vi "(A) Test (SubVI).vi"(0 "References IN":T1, 11 "Initialize":bool, 13 "Strain OK?":bool=TRUE) -> (8 "STOP-PROGRAM":bool, 15 "Step Number":i32)   [LabVIEW 2010]
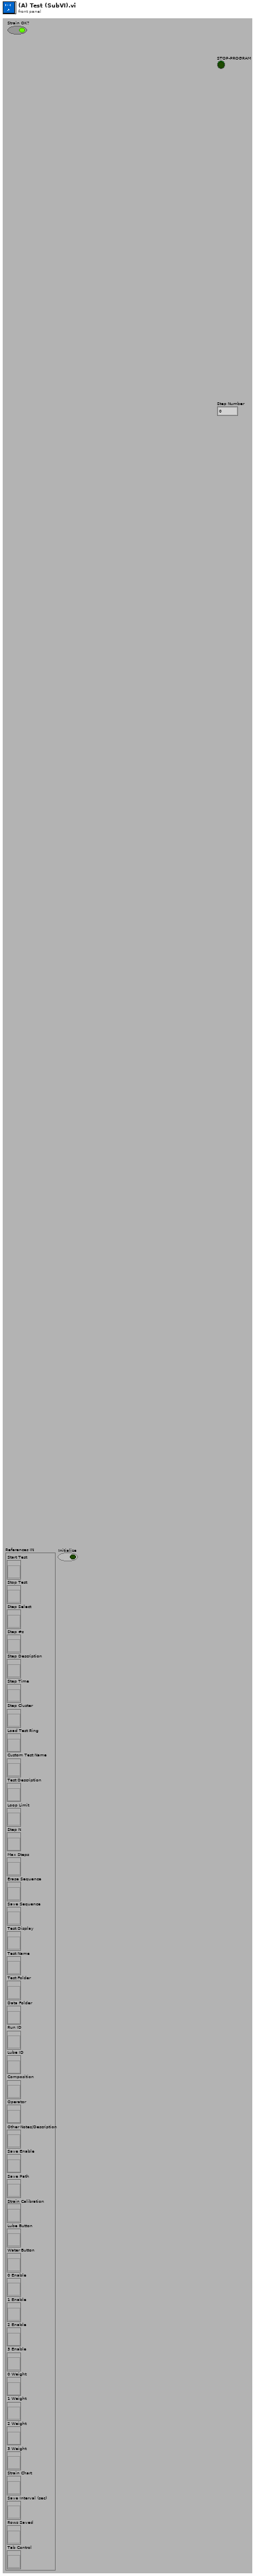
[diagram p1: front panel]
types:
  T1 = cluster{"Start Test":refnum<vi>, "Stop Test":refnum<vi>, "Step Select":refnum<vi>, "Step #s":refnum<vi>, "Step Description":refnum<vi>, "Step Time":refnum<vi>, "Step Cluster":refnum<vi>, "Load Test Ring":refnum<vi>, "Custom Test Name":refnum<vi>, "Test Description":refnum<vi>, "Loop Limit":refnum<vi>, "Step N":refnum<vi>, "Max Steps":refnum<vi>, "Erase Sequence":refnum<vi>, "Save Sequence":refnum<vi>, "Test Display":refnum<vi>, "Test Name":refnum<vi>, "Test Folder":refnum<vi>, "Data Folder":refnum<vi>, "Run ID":refnum<vi>, "Lube ID":refnum<vi>, "Composition":refnum<vi>, "Operator":refnum<vi>, "Other Notes/Description":refnum<vi>, "Save Enable":refnum<vi>, "Save Path":refnum<vi>, "Strain Calibration":refnum<vi>, "Lube Button":refnum<vi>, "Water Button":refnum<vi>, "0 Enable":refnum<vi>, "1 Enable":refnum<vi>, "2 Enable":refnum<vi>, "3 Enable":refnum<vi>, "0 Weight":refnum<vi>, "1 Weight":refnum<vi>, "2 Weight":refnum<vi>, "3 Weight":refnum<vi>, "Strain Chart":refnum<vi>, "Save Interval (sec)":refnum<vi>, "Rows Saved":refnum<vi>, "Tab Control":refnum<vi>}
  T2 = cluster{"Step Time Unit":u16, "Step End Action":u16, "Relay1":bool, "Relay2":bool}[]
  T3 = cluster{"Step Description":string, "Step Time Target":dbl, "Step Time Unit":u16, "Step End Action":u16}
  T4 = cluster{"Step Time Unit":u16, "Step End Action":u16, "Relay1":bool, "Relay2":bool}
  T5 = enum8{"Enabled", "Disabled", "Disabled and Grayed Out"}
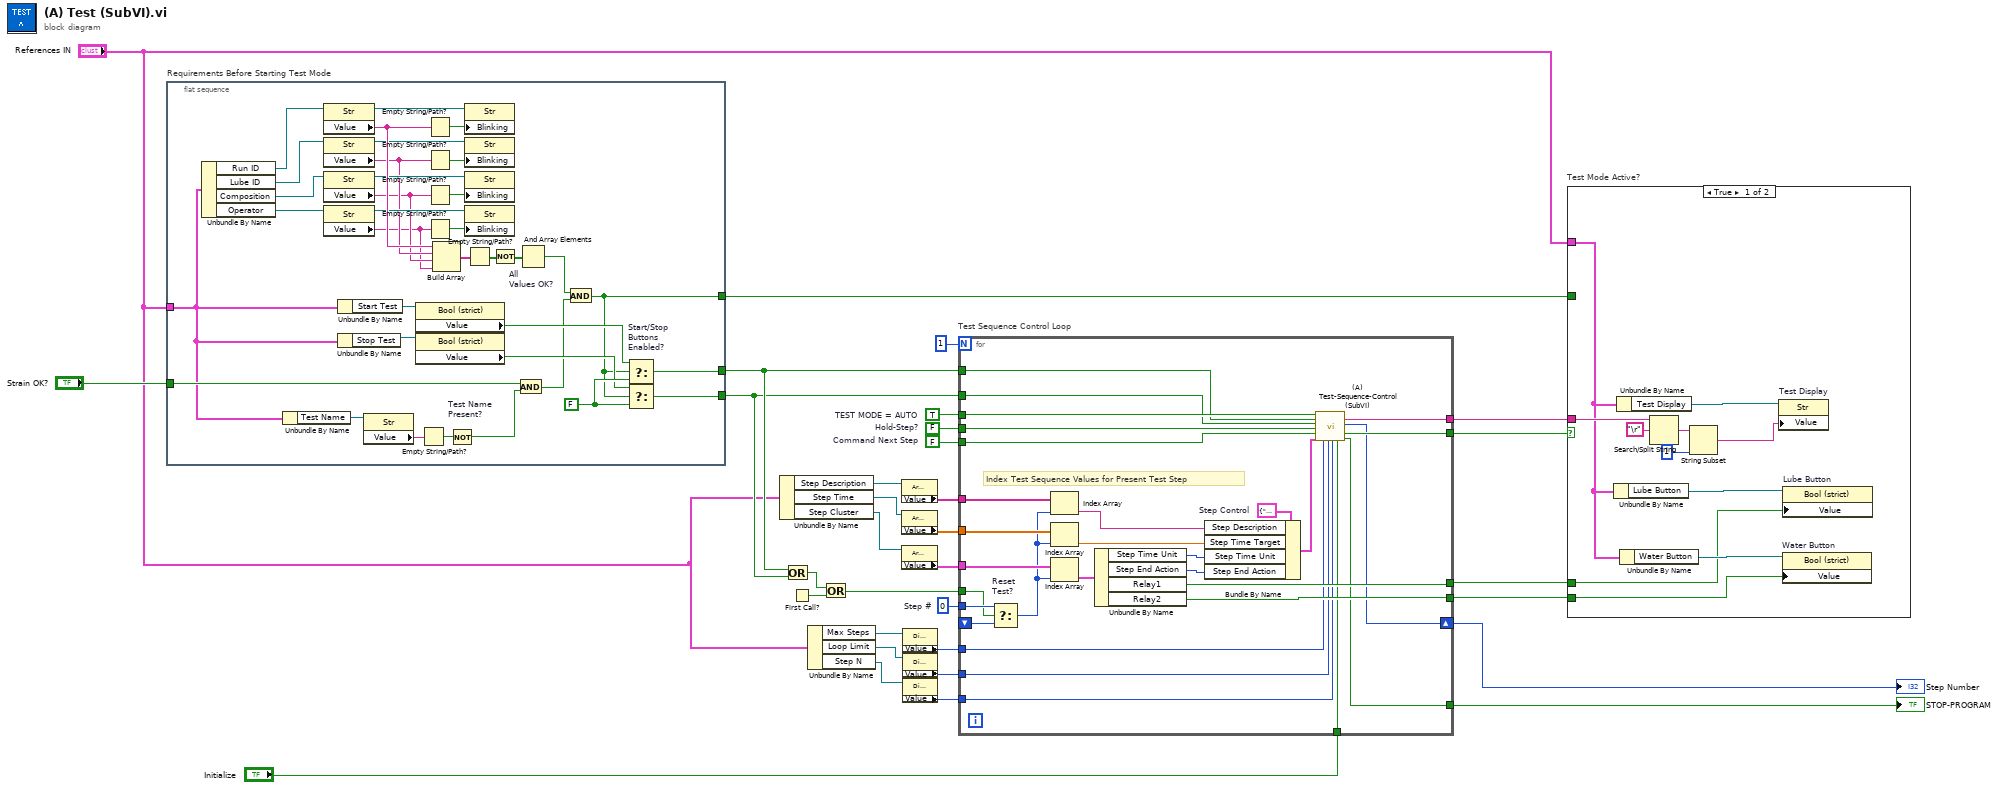
[diagram p0: block diagram]
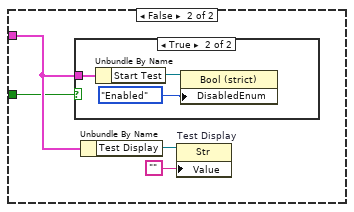
[diagram p2: hidden frame]
diagram:
  w29 = 0  # Step #
  w22 = FALSE  # Command Next Step
  w21 = FALSE  # Hold-Step?
  w20 = TRUE  # TEST MODE = AUTO
  n1 = flat-sequence "Requirements Before Starting Test Mode" {
    tunnel: "Strain OK?" -> [w56]
    tunnel: [w62] -> w32
    tunnel: [w61] -> w4
    tunnel: "References IN" -> [w37]
    tunnel: [w33] -> w2
    frame #0 {
      w65 = FALSE
      n2 = Unbundle By Name(w37) -> ("Run ID"=w53:refnum<vi>, "Lube ID"=w46:refnum<vi>, "Composition"=w43:refnum<vi>, "Operator"=w40:refnum<vi>)
      n3 = Unbundle By Name(w37) -> ("Test Name"=w60:refnum<vi>)
      n4 = property class="Str"(reference=w53) -> (reference out=w54:refnum<vi>, "Value"=w55:string)  [unwired: 1 in, 1 out]
      n5 = property class="Str"(reference=w46) -> (reference out=w47:refnum<vi>, "Value"=w39:string)  [unwired: 1 in, 1 out]
      n6 = property class="Str"(reference=w43) -> (reference out=w44:refnum<vi>, "Value"=w38:string)  [unwired: 1 in, 1 out]
      n7 = property class="Str"(reference=w40) -> (reference out=w41:refnum<vi>, "Value"=w36:string)  [unwired: 1 in, 1 out]
      n8 = Unbundle By Name(w37) -> ("Start Test"=w67:refnum<vi>)
      n9 = Unbundle By Name(w37) -> ("Stop Test"=w66:refnum<vi>)
      n10 = property class="Str"(reference=w60) -> ("Value"=w59:string)  [unwired: 1 in, 2 out]
      n11 = property class="Bool (strict)"(reference=w67) -> ("Value"=w64:bool)  [unwired: 1 in, 2 out]
      n12 = property class="Bool (strict)"(reference=w66) -> ("Value"=w63:bool)  [unwired: 1 in, 2 out]
      n13 = Empty String/Path?(string/path=w59) -> (empty?=w58:bool)
      n14 = Empty String/Path?(string/path=w55) -> (empty?=w49:bool)
      n15 = Empty String/Path?(string/path=w39) -> (empty?=w48:bool)
      n16 = Empty String/Path?(string/path=w38) -> (empty?=w45:bool)
      n17 = Empty String/Path?(string/path=w36) -> (empty?=w42:bool)
      n18 = Build Array(w55, w39, w38, w36) -> (w50:string[])
      n19 = Not "Test Name\nPresent?"(x=w58) -> (.not. x?=w57:bool)
      n20 = property class="Str"(reference=w54, "Blinking"=w49) -> ()  [unwired: 1 in, 2 out]
      n21 = property class="Str"(reference=w47, "Blinking"=w48) -> ()  [unwired: 1 in, 2 out]
      n22 = property class="Str"(reference=w44, "Blinking"=w45) -> ()  [unwired: 1 in, 2 out]
      n23 = property class="Str"(reference=w41, "Blinking"=w42) -> ()  [unwired: 1 in, 2 out]
      n24 = Empty String/Path?(string/path=w50) -> (empty?=w52:bool[])
      n25 = Not(x=w52) -> (.not. x?=w51:bool[])
      n26 = And(x=w56, y=w57) -> (x .and. y?=w35:bool)
      n27 = And Array Elements "All\nValues OK?"(Boolean array=w51) -> (logical AND=w34:bool)
      n28 = And(x=w34, y=w35) -> (x .and. y?=w33:bool)
      n29 = Select "Start/Stop\nButtons \nEnabled?"(t=w64, s=w33, f=w65) -> (s? t:f=w62:bool)
      n30 = Select(t=w63, s=w33, f=w65) -> (s? t:f=w61:bool)
    }
  }
  n31 = Unbundle By Name("References IN") -> ("Step Description"=w16:refnum<vi>, "Step Time"=w14:refnum<vi>, "Step Cluster"=w12:refnum<vi>)
  n32 = Or(x=w32, y=w4) -> (x .or. y?=w23:bool)
  n33 = First Call?() -> (First Call?: T/F=w24:bool)
  n34 = Unbundle By Name("References IN") -> ("Max Steps"=w19:refnum<vi>, "Loop Limit"=w18:refnum<vi>, "Step N"=w17:refnum<vi>)
  n35 = Or(x=w23, y=w24) -> (x .or. y?=w30:bool)
  n36 = property class="Arr (strict)"(reference=w16) -> ("Value"=w15:string[])  [unwired: 1 in, 2 out]
  n37 = property class="Arr (strict)"(reference=w14) -> ("Value"=w13:dbl[])  [unwired: 1 in, 2 out]
  n38 = property class="Arr (strict)"(reference=w12) -> ("Value"=w11:T2)  [unwired: 1 in, 2 out]
  n39 = property on="Max Steps" class="DigNum (strict)"(reference=w19) -> ("Value"=w8:i32)  [unwired: 1 in, 2 out]
  n40 = property on="Loop Limit" class="DigNum (strict)"(reference=w18) -> ("Value"=w26:i32)  [unwired: 1 in, 2 out]
  n41 = property on="Step N" class="DigNum (strict)"(reference=w17) -> ("Value"=w27:i32)  [unwired: 1 in, 2 out]
  n42 = for "Test Sequence Control Loop" {
    N: 1 -> [_]
    tunnel: w20 -> [w92]
    tunnel: w21 -> [w91]
    tunnel: w22 -> [w90]
    tunnel: w32 -> [w89]
    tunnel: w4 -> [w88]
    tunnel: "Initialize" -> [w93]
    tunnel: w26 -> [w87]
    tunnel: w27 -> [w86]
    tunnel: w29 -> [w85]
    tunnel: w30 -> [w84]
    shift-right: [w68] -> w6
    shift-left: _ -> [w83]
    tunnel: [w81] -> w31
    tunnel: [w94] -> w3
    tunnel: [w82] -> w7
    tunnel: w15 -> [w73]
    tunnel: w13 -> [w75]
    tunnel: w11 -> [w77]
    tunnel: [w96] -> w10
    tunnel: [w95] -> w9
    tunnel: w8 -> [w70]
    w71 = T3 {"Step Description"="Description", "Step Time Target"=10.0, "Step Time Unit"=0, "Step End Action"=0}  # Step Control
    # "Index Test Sequence Values for Present Test Step"
    n43 = Select "Reset\nTest?"(t=w85, s=w84, f=w83) -> (s? t:f=w69:i32)
    n44 = Index Array(array=w73, index=w69) -> (element=w72:string)
    n45 = Index Array(array=w75, index=w69) -> (element=w74:dbl)
    n46 = Index Array(array=w77, index=w69) -> (element=w76:T4)
    n47 = Unbundle By Name(w76) -> ("Step Time Unit"=w79:u16, "Step End Action"=w78:u16, "Relay1"=w96:bool, "Relay2"=w95:bool)
    n48 = Bundle By Name(cluster=w71, "Step Description"=w72, "Step Time Target"=w74, "Step Time Unit"=w79, "Step End Action"=w78) -> (w80:T3)
    n49 = call "(A) Test-Sequence-Control (SubVI).vi"("TEST MODE"=w92, "START"=w89, "STOP"=w88, "Hold-Step?"=w91, "Command Next Step"=w90, "Step Control"=w80, "Step # Limit"=w70, "Loop # Limit"=w87, "Step N"=w86, "Initialize"=w93) -> ("Display"=w82:string, "Step Number"=w68:i32, "TEST MODE ACTIVE?"=w81:bool, "STOP-PROGRAM"=w94:bool)  [unwired: 4 in, 2 out]
  }
  "Step Number" <- w6
  "STOP-PROGRAM" <- w3
  n50 = case "Test Mode Active?" shown="True" w31 {
    tunnel: w10 -> [w98 _]
    tunnel: w9 -> [w107 _]
    tunnel: w7 -> [w102 _]
    tunnel: "References IN" -> [w97 w109]
    tunnel: w2 -> [_ w108]
    frame True {
      n51 = Unbundle By Name(w97) -> ("Lube Button"=w105:refnum<vi>)
      n52 = Unbundle By Name(w97) -> ("Test Display"=w106:refnum<vi>)
      n53 = Unbundle By Name(w97) -> ("Water Button"=w104:refnum<vi>)
      n54 = Search/Split String(string=w102, search string/char (-)="\r") -> (match + rest of string=w101:string)  [unwired: 1 in, 2 out]
      n55 = String Subset(string=w101, offset (0)=1) -> (substring=w99:string)  [unwired: 1 in]
      n56 = property on="Test Display" class="Str"(reference=w106, "Value"=w99) -> ()  [unwired: 1 in, 2 out]
      n57 = property on="Water Button" class="Bool (strict)"(reference=w104, "Value"=w107) -> ()  [unwired: 1 in, 2 out]
      n58 = property on="Lube Button" class="Bool (strict)"(reference=w105, "Value"=w98) -> ()  [unwired: 1 in, 2 out]
    }
    frame False {
      n59 = case shown="True" w108 {
        tunnel: w109 -> [_ w114]
        frame False {
        }
        frame True {
          n60 = Unbundle By Name(w114) -> ("Start Test"=w112:refnum<vi>)
          n61 = property class="Bool (strict)"(reference=w112, "DisabledEnum"=T5."Enabled" ("Disabled")) -> ()  [unwired: 1 in, 2 out]
        }
      }
      n62 = Unbundle By Name(w109) -> ("Test Display"=w110:refnum<vi>)
      n63 = property on="Test Display" class="Str"(reference=w110, "Value"="") -> ()  [unwired: 1 in, 2 out]
    }
  }
